vi "Create Path.vi"() -> (0 "Login path":path)   [LabVIEW 2012]
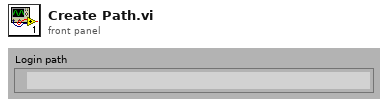
[diagram p1: front panel]
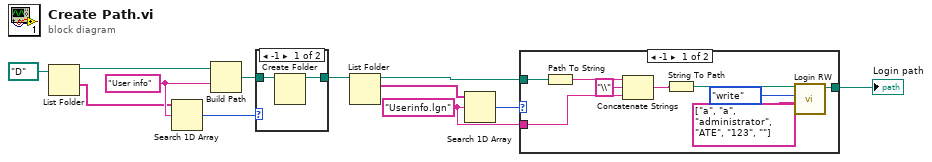
[diagram p0: block diagram]
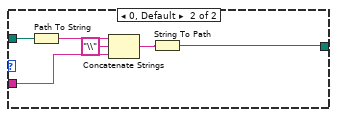
[diagram p3: hidden frame]
diagram:
  w10 = "User info" ("element")
  w5 = "Userinfo.lgn" ("element")
  n1 = List Folder(path=path "D:/" ("base path")) -> (path out=w1:path, folder names=w2:string[])  [unwired: 3 in, 2 out]
  n2 = Search 1D Array(1D array=w2, element=w10) -> (index of element=w9:i32)  [unwired: 1 in]
  n3 = Build Path(base path=w1, name or relative path=w10) -> (appended path=w11:path)
  n4 = case shown="-1" w9 {
    tunnel: [w14 w15] -> w6
    tunnel: w11 -> [w13 w15]
    frame -1 {
      n5 = Create Folder(path (use dialog)=w13) -> (created path=w14:path)  [unwired: 2 in, 2 out]
    }
    frame 0, Default {
    }
  }
  n6 = List Folder(path=w6) -> (path out=w7:path, filenames=w8:string[])  [unwired: 3 in, 2 out]
  n7 = Search 1D Array(1D array=w8, element=w5) -> (index of element=w12:i32)  [unwired: 1 in]
  n8 = case shown="-1" w12 {
    tunnel: w7 -> [w22 w27]
    tunnel: w5 -> [w19 w26]
    tunnel: [w16 w25] -> w4
    frame -1 {
      n9 = Path To String(path=w22) -> (string=w21:string)
      n10 = Concatenate Strings(w21, "\\" ("string"), w19) -> (w18:string)
      n11 = String To Path(string=w18) -> (path=w17:path)
      n12 = call "Login RW.vi"("Table in"=string[][] [["a", "a", "administrator"], ["ATE", "123", ""]], "Enum"=enum16{"write", "read"}."write", "Path in"=w17) -> ("Path out"=w16:path)  [unwired: 6 in, 2 out]
    }
    frame 0, Default {
      n13 = Path To String(path=w27) -> (string=w30:string)
      n14 = Concatenate Strings(w30, "\\" ("string"), w26) -> (w28:string)
      n15 = String To Path(string=w28) -> (path=w25:path)
    }
  }
  "Login path" <- w4
